vi "arrayRowCols.vi"(3 "imageArray":i16[][](array[numeric])) -> (0 "rows":i32, 1 "cols":i32)   [LabVIEW 2021]
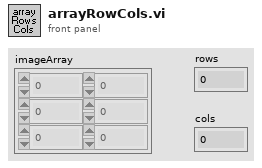
[diagram p1: front panel]
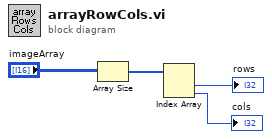
[diagram p0: block diagram]
diagram:
  n1 = Array Size(array="imageArray") -> (size(s)=w3:i32[])
  n2 = Index Array(array=w3) -> (element #1=→"rows":i32, element #2=→"cols":i32)  [unwired: 2 in]
